vi "Active Element.vi"(8 "error in (no error)":errorcluster, 11 "Test Configs In":T1) -> (0 "error out":errorcluster, 2 "Active Test":string, 3 "Test Configs Out":T1)   [LabVIEW 2015]
doc: "Determine which array index is currently being viewed."
uses:
  Type Defs/Sequence Parameters Ref.ctl
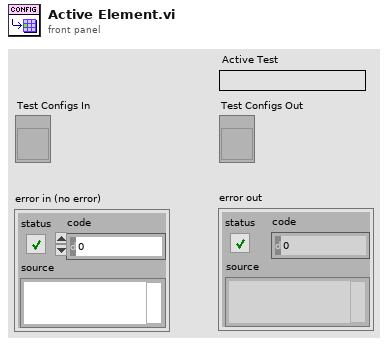
[diagram p1: front panel]
types:
  T1 = typedef "Sequence Parameters Ref.ctl" = refnum<vi>
  T2 = typedef "Sequence Parameters.ctl" = cluster{"Test Name":string, "Target":T3, "Host IP Address":string, "Target IP Address":string, "Shared Variable Host":enum16{"Target", "Host"}, "Shared Variable Writer":enum16{"Target", "Host"}, "Variable Data Type":T4, "# of Variables per Library":u16, "Update Rate (Hz)":dbl, "Read Rate (Hz)":dbl, "Floor":u32, "Ceiling":u32, "Delta":u32}
  T3 = typedef "Target Type.ctl" = enum16{"cRIO-9012", "cRIO-9014", "cRIO-9022", "cRIO-9023", "cRIO-9024", "cRIO-9025", "cRIO-9068", "cRIO-9073", "cRIO-9074", "cRIO-9075", "cRIO-9076", "cRIO-9081", "cRIO-9082", "myRIO-1900", "myRIO-1950", "PXI-8101", "PXI-8115", "PXI-8119", "PXI-8820", "PXIe-8100", "PXIe-8101", "PXIe-8133", "PXIe-8135", "PXIe-8820", "sbRIO-9605", "sbRIO-9606", "sbRIO-9623", "sbRIO-9626", "sbRIO-9633", "sbRIO-9636", "Unlisted (Linux-RT)", "Unlisted (PharLap)", "Unlisted (VxWorks)", "Windows Target"}
  T4 = typedef "Variable Data Type.ctl" = enum16{"U8", "U16", "U32", "U64", "I8", "I16", "I32", "I64", "Single", "Double", "Boolean", "String"}
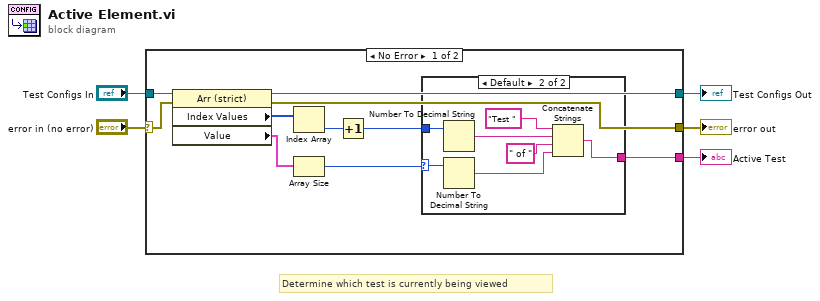
[diagram p0: block diagram]
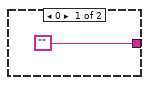
[diagram p2: hidden frame]
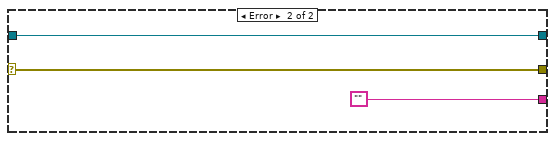
[diagram p3: hidden frame]
diagram:
  # "Determine which test is currently being viewed"
  n1 = case shown="No Error" "error in (no error)" {
    selector: "error in (no error)" -> [w14 w25]
    tunnel: "Test Configs In" -> [w15 w26]
    tunnel: [w8 w26] -> w2
    tunnel: [w7 w25] -> w3
    tunnel: [w11 ""] -> w1
    frame No Error {
      n2 = property class="Arr (strict)"(reference=w15, error in=w14) -> (reference out=w8:T1, error out=w7:errorcluster, "Index Values"=w13:u32[], "Value"=w12:T2[])
      n3 = Index Array(array=w13) -> (element=w9:u32)  [unwired: 1 in]
      n4 = Array Size(array=w12) -> (size(s)=w6:i32)
      n5 = Increment(x=w9) -> (x+1=w10:u32)
      n6 = case shown="Default" w6 {
        selector: w6 -> [_ w17]
        tunnel: ["" w19] -> w11
        tunnel: w10 -> [_ w18]
        frame 0 {
        }
        frame Default {
          n7 = Number To Decimal String(number=w18) -> (decimal integer string=w22:string)  [unwired: 1 in]
          n8 = Number To Decimal String(number=w17) -> (decimal integer string=w20:string)  [unwired: 1 in]
          n9 = Concatenate Strings("Test ", w22, " of ", w20) -> (w19:string)
        }
      }
    }
    frame Error {
    }
  }
  "Test Configs Out" <- w2
  "error out" <- w3
  "Active Test" <- w1
